vi "Average RF Hammers.vi"(4 "Record":waveform(dbl)[](array[waveform])) -> (0 "RF Pulse is Hammer":bool[](array[boolean]), 1 "RF Pulse Start Indicies":u32[](array[numeric]), 2 "Waveform Graph":waveform(dbl)[](graph))   [LabVIEW 2013]
panel:
  out "Integrations":dbl[](array[numeric])
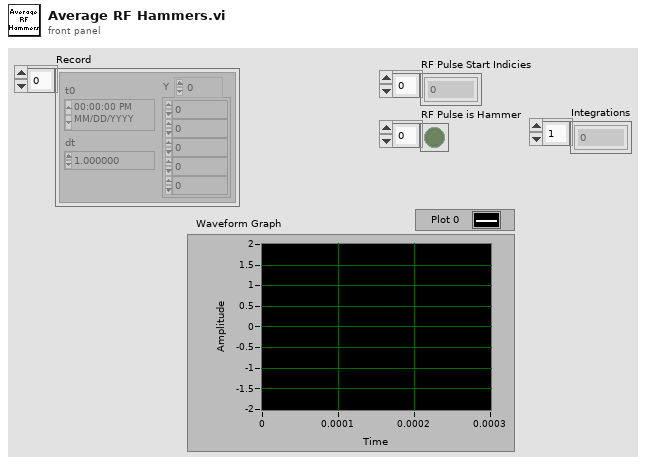
[diagram p1: front panel]
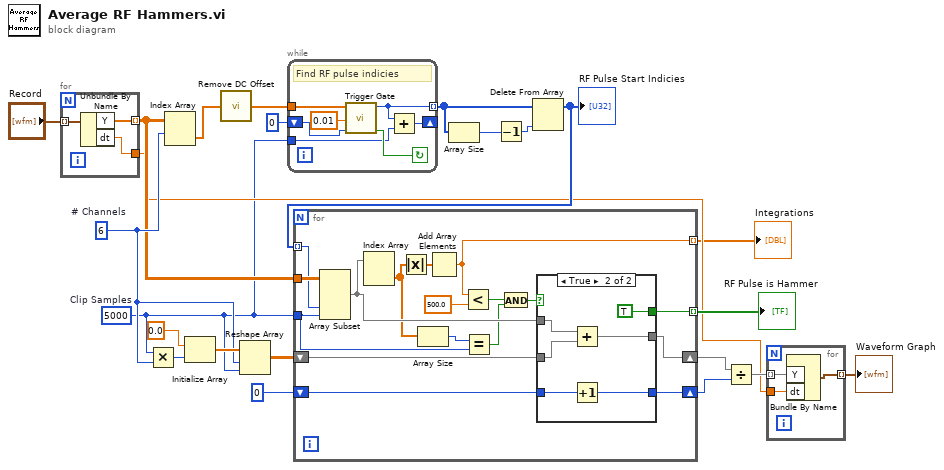
[diagram p0: block diagram]
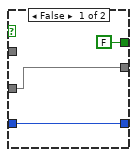
[diagram p2: hidden frame]
diagram:
  w4 = 5000  # Clip Samples
  w14 = 6  # # Channels
  n1 = for {
    tunnel: "Record" -> [w26] mode=indexing
    tunnel: [w25] -> w8 mode=indexing
    tunnel: [w24] -> w5
    n2 = Unbundle By Name(w26) -> ("Y"=w25:dbl[], "dt"=w24:dbl)
  }
  n3 = Multiply(x=w4, y=w14) -> (x*y=w17:i32)
  n4 = Index Array(array=w8, index (row)=w14) -> (element=w3:dbl[])  [unwired: 1 in]
  n5 = Initialize Array(0.0 ("y"), w17) -> (w15:dbl[])
  n6 = call "Remove DC Offset.vi"("Signal"=w3) -> ("Processed Signal"=w2:dbl[])  [unwired: 4 in]
  n7 = Reshape Array(w15, w14, w4) -> (w13:dbl[][])
  n8 = while {
    tunnel: w2 -> [w32]
    tunnel: [w29] -> w22 mode=indexing
    shift-right: [w27] -> _
    shift-left: u32 0 ("Stop") -> [w31]
    tunnel: w4 -> [w28]
    stop <- w30 continue-if-true
    # "Find RF pulse indicies"
    n9 = call "Trigger Gate.vi"("Offset (0)"=w31, "Threshold"=0.01, "Waveform"=w32) -> ("Satisfied"=w30:bool, "Start"=w29:u32)  [unwired: 6 in, 1 out]
    n10 = Add(x=w29, y=w28) -> (x+y=w27:u32)
  }
  n11 = Array Size(array=w22) -> (size(s)=w21:i32)
  n12 = Decrement(x=w21) -> (x-1=w20:i32)
  n13 = Delete From Array(array=w22, index=w20) -> (array with subset deleted=w19:u32[])  [unwired: 1 in, 1 out]
  "RF Pulse Start Indicies" <- w19
  n14 = for {
    tunnel: w8 -> [w50]
    tunnel: w19 -> [w49] mode=indexing
    tunnel: w4 -> [w39]
    shift-right: [w45] -> w11
    shift-left: 0 -> [w46]
    shift-right: [w43] -> w12
    shift-left: w13 -> [w44]
    tunnel: [w42] -> w10 mode=indexing
    tunnel: [w41] -> w1 mode=indexing
    n15 = Array Subset(array=w50, index (col)=w49, length (col)=w39) -> (w40:dbl[][])  [unwired: 2 in]
    n16 = Index Array(array=w40) -> (element=w35:dbl[])  [unwired: 2 in]
    n17 = Absolute Value(x=w35) -> (abs(x)=w48:dbl[])
    n18 = Array Size(array=w35) -> (size(s)=w34:i32)
    n19 = Add Array Elements(numeric array=w48) -> (sum=w41:dbl)
    n20 = Less?(x=w41, y=500.0) -> (x < y?=w37:bool)
    n21 = Equal?(x=w34, y=w39) -> (x = y?=w36:bool)
    n22 = And(x=w37, y=w36) -> (x .and. y?=w38:bool)
    n23 = case shown="True" w38 {
      tunnel: w40 -> [_ w57]
      tunnel: w46 -> [w52 w59]
      tunnel: [w52 w58] -> w45
      tunnel: w44 -> [w53 w56]
      tunnel: [w53 w55] -> w43
      tunnel: [FALSE TRUE] -> w42
      frame False {
      }
      frame True {
        n24 = Add(x=w57, y=w56) -> (x+y=w55:dbl[][])
        n25 = Increment(x=w59) -> (x+1=w58:i32)
      }
    }
  }
  "RF Pulse is Hammer" <- w10
  "Integrations" <- w1
  n26 = Divide(x=w12, y=w11) -> (x/y=w7:dbl[][])
  n27 = for {
    tunnel: w7 -> [w62] mode=indexing
    tunnel: [w61] -> w6 mode=indexing
    tunnel: w5 -> [w60]
    n28 = Bundle By Name("Y"=w62, "dt"=w60) -> (w61:waveform(dbl))  [unwired: 1 in]
  }
  "Waveform Graph" <- w6
